vi "Valid.vi"(11 "gesture in":refnum<class "Gesture.lvclass">) -> (2 "valid":bool)   [LabVIEW 2019, in "Gesture.lvclass"]
doc: "Retrieve whether or not this is a valid gesture."
uses:
  Gesture.lvclass
  Gesture Enum.ctl
  Gesture.lvclass/Gesture.ctl
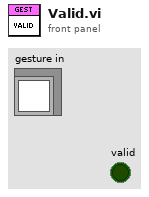
[diagram p1: front panel]
types:
  T1 = typedef "Gesture.lvclass/Gesture Enum.ctl" = enum16{"None", "Stop", "Tap", "Press", "Pan Start", "Pan Continue", "Pan End", "Pinch Open", "Pinch Close", "Double Tap"}
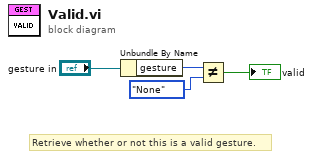
[diagram p0: block diagram]
diagram:
  # "Retrieve whether or not this is a valid gesture."
  n1 = Unbundle By Name("gesture in") -> ("gesture"=w3:T1)
  n2 = Not Equal?(x=w3, y=Gesture_Enum."None") -> (x != y?=→"valid":bool)
